vi "simple_FFT.vi"(1 "x(t)":dbl[](array[numeric])) -> (0 "X(w)":cdb[](array[numeric]))   [LabVIEW 2020, in "dsdll.lvlib"]
doc: "Simple script based FFT. Uses Cooley-Tukey radix-2 Decimation-In-Time algorithm. Will work only for data sets of length N = 2^M, where M is integer."
uses:
  dsdll.lvlib
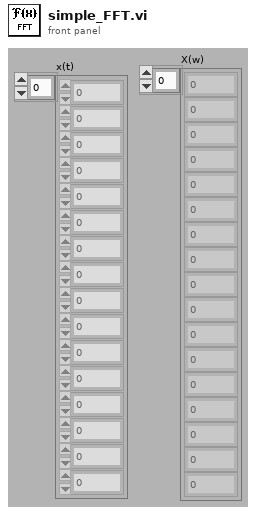
[diagram p1: front panel]
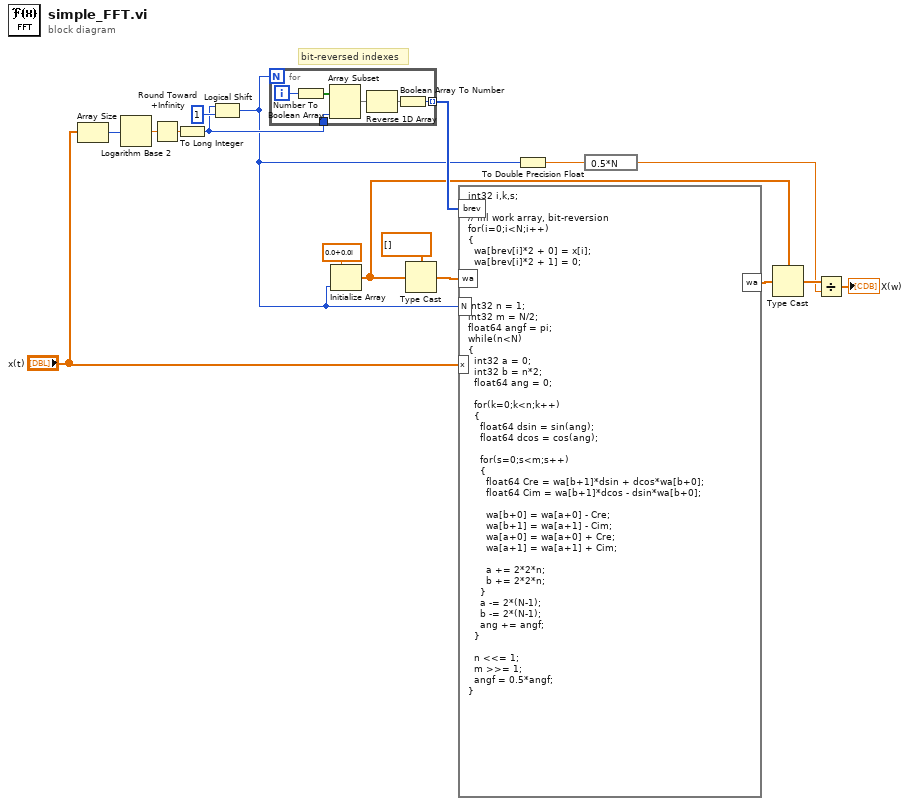
[diagram p0: block diagram]
diagram:
  # "bit-reversed indexes"
  n1 = Array Size(array="x(t)") -> (size(s)=w7:i32)
  n2 = Logarithm Base 2(1:w7) -> (0:w12:dbl)
  n3 = Round Toward +Infinity(x=w12) -> (ceil(x): smallest int >= x=w11:dbl)
  n4 = To Long Integer(number=w11) -> (32bit integer=w9:i32)
  n5 = Logical Shift(y=w9, x=u32 1) -> (x << y=w4:u32)
  n6 = for {
    N: w4 -> [_]
    tunnel: w9 -> [w22]
    tunnel: [w19] -> w16 mode=indexing
    i -> [w18]
    n7 = Number To Boolean Array(number=w18) -> (Boolean array=w23:bool[])
    n8 = Array Subset(array=w23, length=w22) -> (w21:bool[])  [unwired: 1 in]
    n9 = Reverse 1D Array(array=w21) -> (reversed array=w20:bool[])
    n10 = Boolean Array To Number(Boolean array=w20) -> (number=w19:u32)
  }
  n11 = Initialize Array(cdb 0.0+0.0i ("element"), w4) -> (w13:cdb[])
  n12 = Type Cast(type=dbl[] [], x=w13) -> (*(type *) &x=w15:dbl[])
  n13 = formula code="int32 i,k,s;\n\n// fill work array, bit-reversion\nfor(i=0;i<N;i++)\n{\n  wa[brev[i]*2 + 0] = x[i];\n  wa[brev[i]*2 + 1] = 0;\n}\n\n\nint32 n = 1;\nint32 m = N/2;\nfloat64 angf = pi;\nwhile(n<N)\n{\n  int32 a = 0;\n  int32 b = n*2;\n  float64 ang = 0;\n\n  for(k=0;k<n;k++)\n  {\n    float64 dsin = sin(ang);\n    float64 dcos = cos(ang);\n\n    for(s=0;s<m;s++)\n    {\n      float64 Cre = wa[b+1]*dsin + dcos*wa[b+0];\n      float64 Cim = wa[b+1]*dcos - dsin*wa[b+0];\n      \n      wa[b+0] = wa[a+0] - Cre;\n      wa[b+1] = wa[a+1] - Cim;\n      wa[a+0] = wa[a+0] + Cre;\n      wa[a+1] = wa[a+1] + Cim;\n      \n      a += 2*2*n;\n      b += 2*2*n;\n    }\n    a -= 2*(N-1);\n    b -= 2*(N-1);\n    ang += angf;\n  }\n\n  n <<= 1;\n  m >>= 1;\n  angf = 0.5*angf;\n}"("x"="x(t)", "N"=w4, "wa"=w15, "brev"=w16) -> ("wa"=w8:dbl[])
  n14 = To Double Precision Float(number=w4) -> (double precision float=w1:dbl)
  n15 = expression code="0.5*N"(w1) -> (w3:dbl)
  n16 = Type Cast(type=w13, x=w8) -> (*(type *) &x=w5:cdb[])
  n17 = Divide(x=w5, y=w3) -> (x/y=→"X(w)":cdb[])
